vi "From String Array.vi"(8 "error in (no error)":errorcluster, 11 "Step Config in":refnum<class "Step Config.lvclass">) -> (0 "error out":errorcluster, 3 "Step Config out":refnum<class "Step Config.lvclass">)   [LabVIEW 2015, in "Step Config.lvclass"]
uses:
  Step Config.lvclass
panel:
  in  "String Array":string[][](array[string])
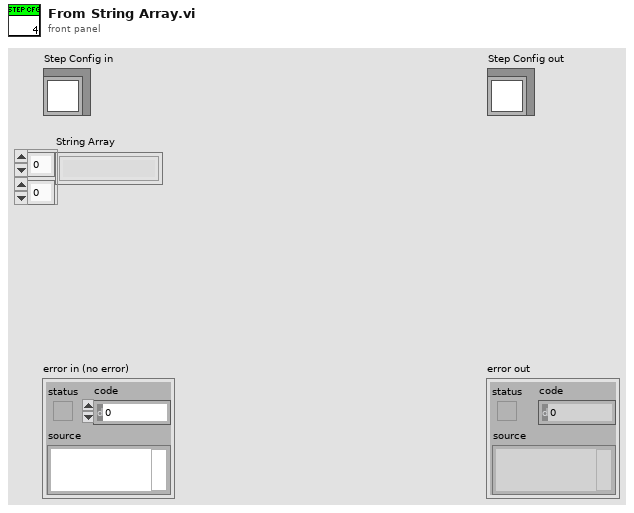
[diagram p1: front panel]
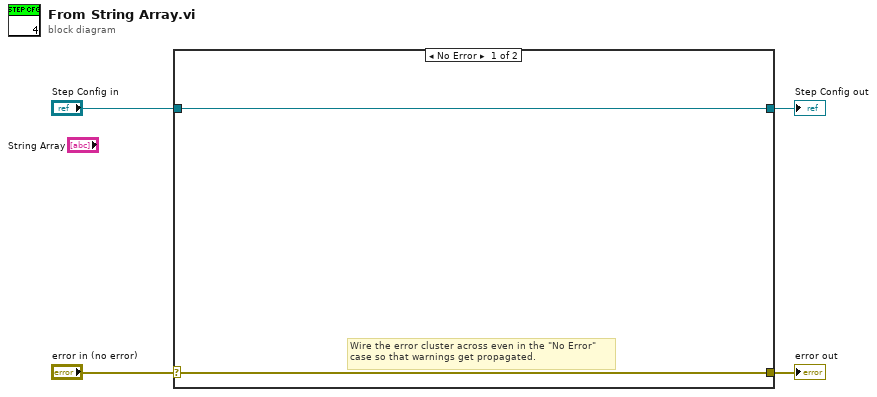
[diagram p0: block diagram]
diagram:
  n1 = case shown="No Error" "error in (no error)" {
    selector: "error in (no error)" -> [w5 w8]
    tunnel: [w5 w8] -> w3
    tunnel: [w6 w7] -> w1
    tunnel: "Step Config in" -> [w6 w7]
    frame No Error {
      # "Wire the error cluster across even in the \"No Error\"\ncase so that warnings get propagated."
    }
    frame Error {
    }
  }
  "error out" <- w3
  "Step Config out" <- w1
